vi "FindParticles.vi"(8 "error in (no error)":errorcluster, 9 "Calibration 2":T4={"Pixel Width (X)"=1.0, "Pixel Height (Y)"=1.0}, 10 "TrackingSettings":T5={"Max Radius"=0, "Threshold"=0.0, "ROI"={"Left"=1, "Top"=1, "Right"=2, "Bottom"=0, "Rotation"=0.0}} {"ROI"."Rotation" format="%.2f"; "ROI"."Left" scale=0.0..1024.0; "ROI"."Right" scale=0.0..1024.0; "Threshold" scale=0.0..255.0}, 11 "?":T2) -> (0 "error out 2":errorcluster, 2 "Centroids 2":dbl[][](array[numeric]), 3 "?":T2)   [LabVIEW 2017, in "ImageAcquisitionLibrary.lvlib"]
uses:
  ImageAcquisitionLibrary.lvlib
  TrackingSettings.ctl
  Settings/Calibration.ctl
  TrackingImages.ctl
  <vilib>/vision/Image Controls.llb/IMAQ Image.ctl
  <vilib>/vision/NI_Vision_Development_Module.lvlib
panel:
  in  "ROI":T1 {"Rotation" format="%.2f"; "Left" scale=0.0..1024.0; "Right" scale=0.0..1024.0}
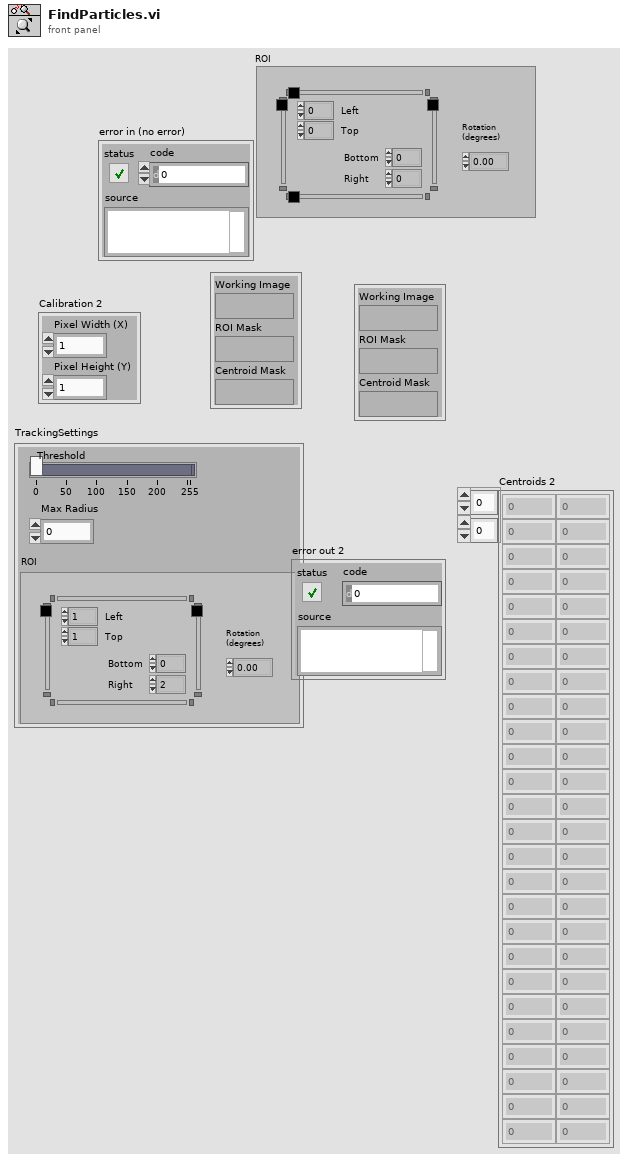
[diagram p1: front panel]
types:
  T1 = typedef "IMAQ Rectangle" = cluster{"Left":i32, "Top":i32, "Right":i32, "Bottom":i32, "Rotation":dbl}
  T2 = typedef "ImageAcquisitionLibrary.lvlib/TrackingImages.ctl" = cluster{"Working Image":T3, "ROI Mask":T3, "Centroid Mask":T3}
  T3 = typedef "IMAQ Image.ctl" = refnum<image>
  T4 = typedef "ImageAcquisitionLibrary.lvlib/Calibration.ctl" = cluster{"Pixel Width (X)":dbl, "Pixel Height (Y)":dbl}
  T5 = typedef "ImageAcquisitionLibrary.lvlib/TrackingSettings.ctl" = cluster{"Max Radius":i32, "Threshold":sgl, "ROI":T1}
  T6 = typedef "IMAQ Circle" = cluster{"Center X":i32, "Center Y":i32, "Inner Radius":i32, "Outer Radius":i32, "Start Angle":dbl, "End Angle":dbl}
  T7 = typedef "Particle Parameters" = i32
  T8 = typedef "ROI Descriptor" = cluster{"Global Rectangle":i32[], "Contours":cluster{"ID":enum32{"External", "Internal"}, "Type":u32, "Coordinates":i32[]}[]}
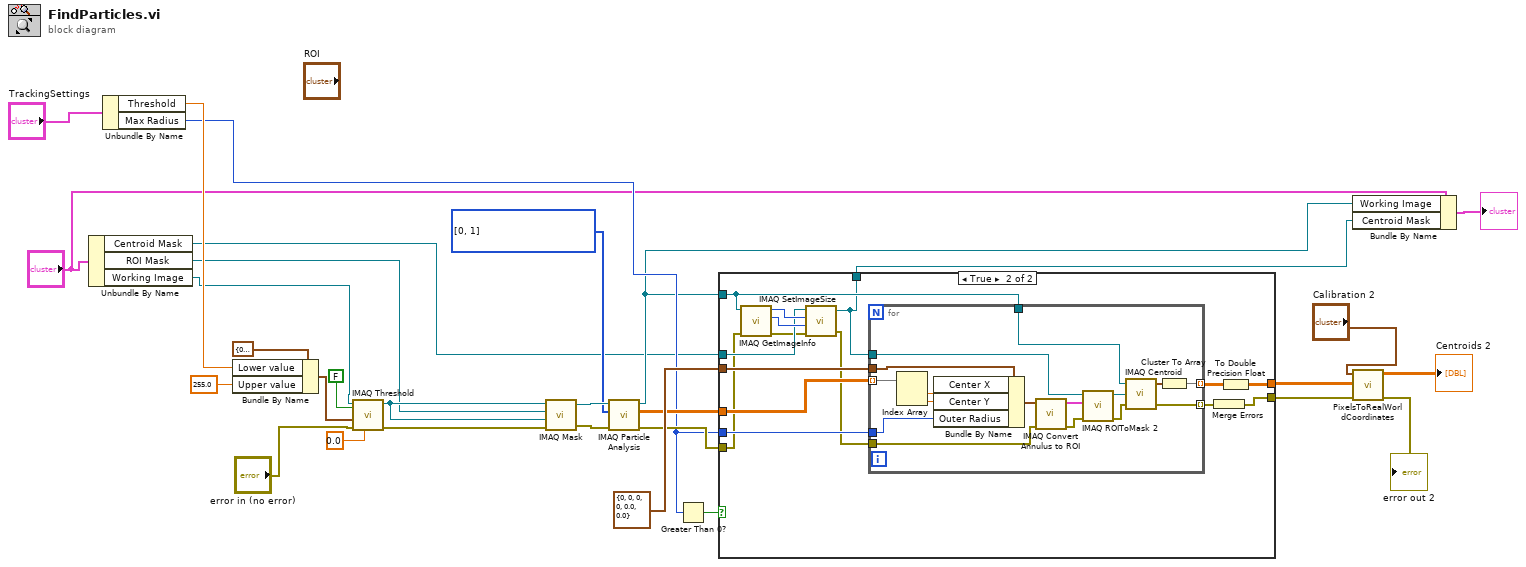
[diagram p0: block diagram]
diagram:
  w21 = T7[] [0, 1] items=["Center of Mass X", "Center of Mass Y", "First Pixel X", "First Pixel Y", "Bounding Rect Left", "Bounding Rect Top", "Bounding Rect Right", "Bounding Rect Bottom", "Max Feret Diameter Start X", "Max Feret Diameter Start Y", "Max Feret Diameter End X", "Max Feret Diameter End Y", "Max Horiz. Segment Length Left", "Max Horiz. Segment Length Right", "Max Horiz. Segment Length Row", "-", "Bounding Rect Width", "Bounding Rect Height", "Bounding Rect Diagonal", "Perimeter", "Convex Hull Perimeter", "Holes' Perimeter", "Max Feret Diameter", "Equivalent Ellipse Major Axis", "Equivalent Ellipse Minor Axis", "Equivalent Ellipse Minor Axis (Feret)", "Equivalent Rect Long Side", "Equivalent Rect Short Side", "Equivalent Rect Diagonal", "Equivalent Rect Short Side (Feret)", "Average Horiz. Segment Length", "Average Vert. Segment Length", "Hydraulic Radius", "Waddel Disk Diameter", "-", "Area", "Holes' Area", "Particle & Holes' Area", "Convex Hull Area", "Image Area", "-", "Number of Holes", "Number of Horiz. Segments", "Number of Vert. Segments", "-", "Orientation", "Max Feret Diameter Orientation", "-", "% Area/Image Area", "% Area/(Particle & Holes' Area)", "Ratio of Equivalent Ellipse Axes", "Ratio of Equivalent Rect Sides", "-", "Elongation Factor", "Compactness Factor", "Heywood Circularity Factor", "Type Factor", "-", "Sum X", "Sum Y", "Sum XX", "Sum XY", "Sum YY", "Sum XXX", "Sum XXY", "Sum XYY", "Sum YYY", "-", "Moment of Inertia XX", "Moment of Inertia XY", "Moment of Inertia YY", "Moment of Inertia XXX", "Moment of Inertia XXY", "Moment of Inertia XYY", "Moment of Inertia YYY", "Norm. Moment of Inertia XX", "Norm. Moment of Inertia XY", "Norm. Moment of Inertia YY", "Norm. Moment of Inertia XXX", "Norm. Moment of Inertia XXY", "Norm. Moment of Inertia XYY", "Norm. Moment of Inertia YYY", "Hu Moment 1", "Hu Moment 2", "Hu Moment 3", "Hu Moment 4", "Hu Moment 5", "Hu Moment 6", "Hu Moment 7"] ("Pixel Measurements")
  n1 = Unbundle By Name("?") -> ("Centroid Mask"=w2:T3, "ROI Mask"=w4:T3, "Working Image"=w5:T3)
  n2 = Unbundle By Name("TrackingSettings") -> ("Threshold"=w28:sgl, "Max Radius"=w10:i32)
  n3 = Bundle By Name(cluster=cluster{"Lower value":sgl, "Upper value":sgl} {"Lower value"=0.0, "Upper value"=0.0} ("Range"), "Lower value"=w28, "Upper value"=sgl 255.0) -> (w26:cluster{"Lower value":sgl, "Upper value":sgl})
  n4 = call "IMAQ Threshold"("Replace Value"=sgl 0.0, "Keep/Replace Value (Replace)"=FALSE, "error in (no error)"="error in (no error)", "Range"=w26, "Image Src"=w5) -> ("error out"=w3:errorcluster, "Image Dst Out"=w6:T3)  [unwired: 5 in]
  n5 = call "IMAQ Mask"("error in (no error)"=w3, "Image Dst"=w6, "Image Mask"=w4, "Image Src"=w6) -> ("error out"=w20:errorcluster, "Image Dst Out"=w22:T3)  [unwired: 1 in]
  n6 = call "IMAQ Particle Analysis"("error in (no error)"=w20, "Pixel Measurements"=w21, "Image"=w22) -> ("error out"=w18:errorcluster, "Particle Measurements (Pixels)"=w16:dbl[][], "Image Out (duplicate)"=w7:T3)  [unwired: 3 in, 3 out]
  n7 = Greater Than 0?(x=w10) -> (x > 0?=w17:bool)
  n8 = case shown="True" w17 {
    tunnel: w2 -> [w31 w38]
    tunnel: T6 {"Center X"=0, "Center Y"=0, "Inner Radius"=0, "Outer Radius"=0, "Start Angle"=0.0, "End Angle"=0.0} ("Annulus") -> [_ w47]
    tunnel: w16 -> [w33 w46]
    tunnel: w10 -> [_ w45]
    tunnel: [w33 w42] -> w11
    tunnel: w18 -> [w32 w36]
    tunnel: [w32 w44] -> w12
    tunnel: w7 -> [_ w41]
    tunnel: [w31 w34] -> w1
    frame False {
    }
    frame True {
      n9 = call "IMAQ GetImageInfo"("error in (no error)"=w36, "Image"=w41) -> ("error out"=w37:errorcluster, "Y Resolution"=w39:i32, "X Resolution"=w40:i32)  [unwired: 2 in, 5 out]
      n10 = call "IMAQ SetImageSize"("error in (no error)"=w37, "Y Resolution"=w39, "X Resolution"=w40, "Image"=w38) -> ("error out"=w35:errorcluster, "Image Out"=w34:T3)  [unwired: 1 in]
      n11 = for {
        tunnel: w46 -> [w64] mode=indexing
        tunnel: [w55] -> w43 mode=indexing
        tunnel: w41 -> [w57]
        tunnel: w34 -> [w59]
        tunnel: [w52] -> w48 mode=indexing
        tunnel: w47 -> [w51]
        tunnel: w45 -> [w50]
        tunnel: w35 -> [w49]
        n12 = Index Array(array=w64) -> (element #1=w62:dbl, element #2=w63:dbl)  [unwired: 2 in]
        n13 = Bundle By Name(cluster=w51, "Center X"=w62, "Center Y"=w63, "Outer Radius"=w50) -> (w61:T6)
        n14 = call "IMAQ Convert Annulus to ROI"("error in (no error)"=w49, "Annulus"=w61) -> ("error out"=w54:errorcluster, "ROI Descriptor"=w60:T8)  [unwired: 7 in]
        n15 = call "IMAQ ROIToMask 2"("error in (no error)"=w54, "ROI Descriptor"=w60, "Image"=w59) -> ("error out"=w53:errorcluster, "Image Out"=w58:T3)  [unwired: 6 in, 1 out]
        n16 = call "IMAQ Centroid"("error in (no error)"=w53, "Image Mask"=w58, "Image"=w57) -> ("error out"=w52:errorcluster, "Centroid"=w56:cluster{"X Centroid":sgl, "Y Centroid":sgl})  [unwired: 1 in]
        n17 = Cluster To Array(cluster=w56) -> (array=w55:sgl[])
      }
      n18 = Merge Errors(w48) -> (w44:errorcluster)
      n19 = To Double Precision Float(number=w43) -> (double precision float=w42:dbl[][])
    }
  }
  n20 = Bundle By Name(cluster="?", "Working Image"=w7, "Centroid Mask"=w1) -> (→"?":T2)
  n21 = call "PixelsToRealWorldCoordinates.vi"("error in (no error)"=w12, "Pixels"=w11, "Calibration 2"="Calibration 2") -> ("error out"=→"error out 2":errorcluster, "Real World Points"=→"Centroids 2":dbl[][])  [unwired: 6 in]
